vi "FORLAB2.vi"() -> ()   [LabVIEW 2015]
uses:
  <vilib>/measure/NI_MABase.lvlib
  <vilib>/Analysis/NI_AALBase.lvlib
  <vilib>/Analysis/3filter.llb/Butterworth Filter (DBL).vi
  <vilib>/Analysis/3filter.llb/Filter Passband Type.ctl
panel:
  in  "Graph Scale":dbl=200.0
  out "Response Time (s)":dbl
  out "Cuttoff Frequency (Hz)":dbl
  in  "stop":bool
  out "Lock-in Signal":waveform(dbl)(graph)
  out "RMS Chart":dbl[](graph)
  out "Reference Signal":waveform(dbl)(graph)
  out "Signal":waveform(dbl)(graph)
  in  "Sample Points":dbl=100.0
  in  "Sampling Rate":dbl=100.0
  in  "Phase (Degrees)":dbl=100.0
  in  "Slider_Offset":dbl(slide) scale=-5.0..5.0
  in  "Slide_Amp":dbl(slide) scale=0.0..5.0
  in  "Frequency (Hz)":dbl=100.0
  # "Amplitude (V)"
  # "Offset (V)"
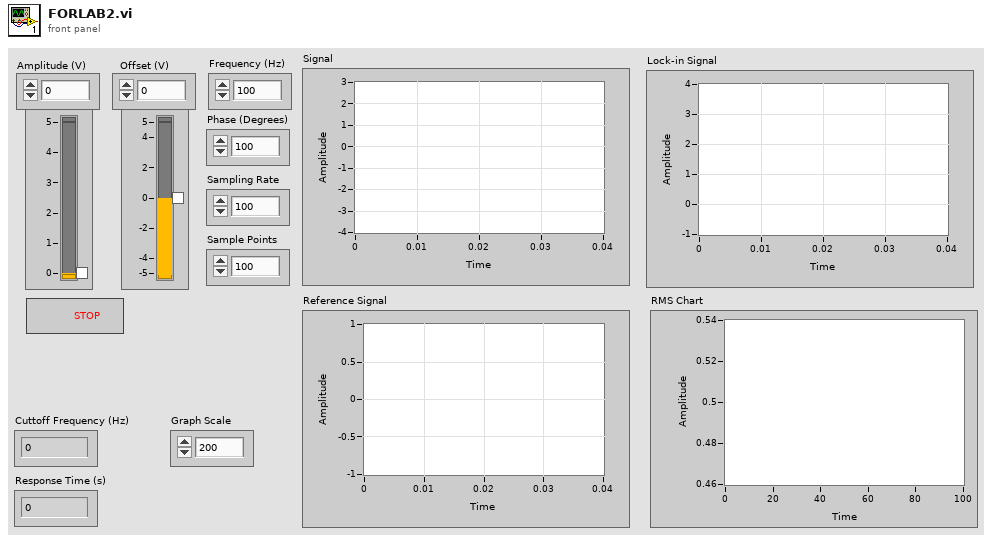
[diagram p1: front panel]
types:
  T1 = cluster{"Sampling Rate":dbl, "Sample Points":dbl}
  T2 = typedef "NI_AALBase.lvlib/Filter Passband Type.ctl" = enum32{"Lowpass", "Highpass", "Bandpass", "Bandstop"}
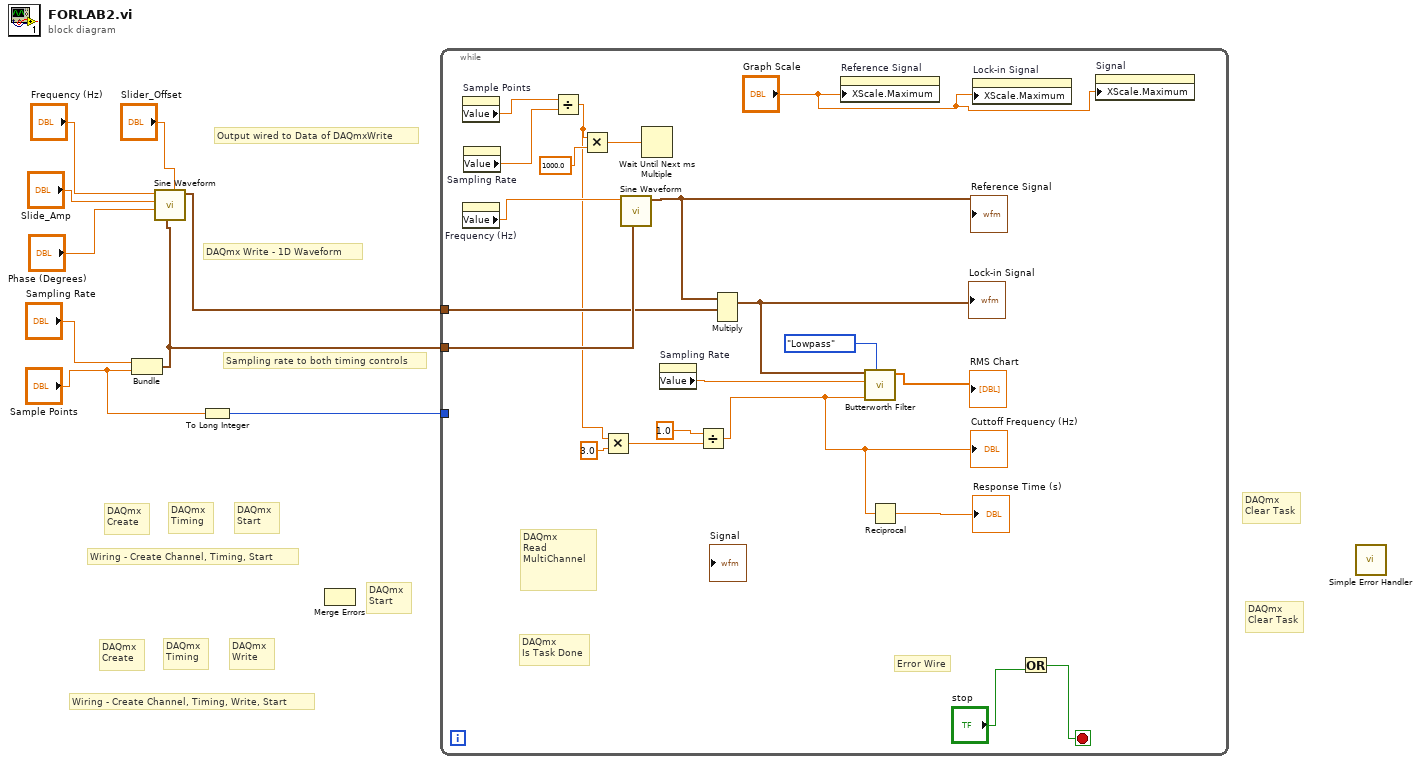
[diagram p0: block diagram]
diagram:
  # "DAQmx\nClear Task"
  # "DAQmx\nClear Task"
  # "DAQmx\nStart"
  # "Sampling rate to both timing controls"
  # "DAQmx\nStart"
  # "DAQmx\nTiming"
  # "DAQmx\nCreate"
  # "DAQmx\nWrite"
  # "DAQmx\nTiming"
  # "DAQmx\nCreate"
  # "Output wired to Data of DAQmxWrite"
  # "Wiring - Create Channel, Timing, Start"
  # "Wiring - Create Channel, Timing, Write, Start"
  # "DAQmx Write - 1D Waveform"
  n1 = Bundle("Sampling Rate"="Sampling Rate", "Sample Points"="Sample Points") -> (w2:T1)  [unwired: 1 in]
  n2 = call <vilib>:"Sine Waveform.vi"("offset"="Slider_Offset", "sampling info"=w2, "phase"="Phase (Degrees)", "amplitude"="Slide_Amp", "frequency"="Frequency (Hz)") -> ("signal out"=w3:waveform(dbl))  [unwired: 5 in, 1 out]
  n3 = To Long Integer(number="Sample Points") -> (32bit integer=w1:i32)
  n4 = Merge Errors() -> ()  [unwired: 2 in, 1 out]
  n5 = while {
    tunnel: w3 -> [w21]
    tunnel: w2 -> [w24]
    tunnel: w1 -> [_]
    stop <- w29 stop-if-true
    # "Error Wire"
    # "DAQmx\nIs Task Done"
    # "DAQmx\nRead\nMultiChannel"
    n6 = property on="Sample Points" class="DigNum (strict)"() -> ("Value"=w27:dbl)  [unwired: 2 in, 2 out]
    n7 = property on="Frequency (Hz)" class="DigNum (strict)"() -> ("Value"=w23:dbl)  [unwired: 2 in, 2 out]
    n8 = property on="Sampling Rate" class="DigNum (strict)"() -> ("Value"=w28:dbl)  [unwired: 2 in, 2 out]
    n9 = Divide(x=w27, y=w28) -> (x/y=w14:dbl)
    n10 = Multiply(x=w14, y=1000.0) -> (x*y=w25:dbl)
    n11 = Multiply(x=w14, y=3.0) -> (x*y=w15:dbl)
    n12 = call <vilib>:"Sine Waveform.vi"("sampling info"=w24, "frequency"=w23) -> ("signal out"=w22:waveform(dbl))  [unwired: 8 in, 1 out]
    "Reference Signal" <- w22
    n13 = Wait Until Next ms Multiple(millisecond multiple=w25) -> ()  [unwired: 1 out]
    n14 = property on="Sampling Rate" class="DigNum (strict)"() -> ("Value"=w18:dbl)  [unwired: 2 in, 2 out]
    n15 = Divide(x=1.0, y=w15) -> (x/y=w11:dbl)
    "Cuttoff Frequency (Hz)" <- w11
    n16 = Multiply(1:w21, 2:w22) -> (0:w19:waveform(dbl))  [unwired: 1 in, 1 out]
    "Lock-in Signal" <- w19
    n17 = property on="Reference Signal" class="WFGraph (strict)"("XScale.Maximum"="Graph Scale") -> ()  [unwired: 2 in, 2 out]
    n18 = call-poly <vilib>:"Butterworth Filter.vi"("filter type"=Filter_Passband_Type."Lowpass", "low cutoff freq: fl"=w11, "sampling freq: fs"=w18, "X"=w19) -> ("Filtered X"=→"RMS Chart":dbl[])  [unwired: 4 in, 1 out]
    n19 = Reciprocal(x=w11) -> (1/x=→"Response Time (s)":dbl)
    n20 = property on="Lock-in Signal" class="WFGraph (strict)"("XScale.Maximum"="Graph Scale") -> ()  [unwired: 2 in, 2 out]
    n21 = Or(y="stop") -> (x .or. y?=w29:bool)  [unwired: 1 in]
    n22 = property on="Signal" class="WFGraph (strict)"("XScale.Maximum"="Graph Scale") -> ()  [unwired: 2 in, 2 out]
  }
  n23 = call <vilib>:"Simple Error Handler.vi"() -> ()  [unwired: 5 in, 5 out]
